vi "P2.vi"() -> ()   [LabVIEW 2019]
panel:
  in  "Stop Button":bool
  out "F":dbl
  in  "C":dbl
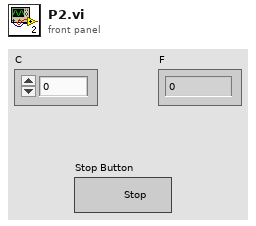
[diagram p1: front panel]
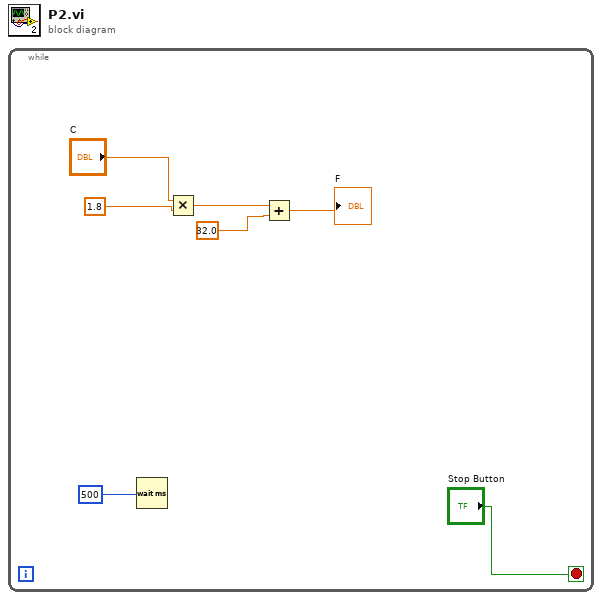
[diagram p0: block diagram]
diagram:
  n1 = while {
    stop <- "Stop Button" stop-if-true
    n2 = Wait (ms)(milliseconds to wait=u32 500 ("millisecond timer value")) -> ()  [unwired: 1 out]
    n3 = Multiply(x="C", y=1.8 ("F")) -> (x*y=w6:dbl)
    n4 = Add(x=w6, y=32.0) -> (x+y=→"F":dbl)
  }
